vi "Generate Calibration Resists.vi"(1 "T Resolution":dbl=0.001 format="%.4f", 2 "End T":dbl=310.0 format="%.2f", 3 "Start T":dbl=1.0 format="%.2f", 4 "# of Points":i32=97) -> (0 "?":dbl[](array[numeric]) format="%.4f")   [LabVIEW 2020]
panel:
  # "Temperatures"
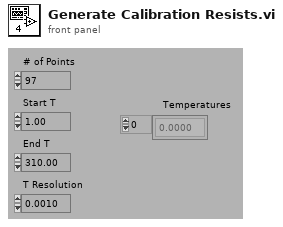
[diagram p1: front panel]
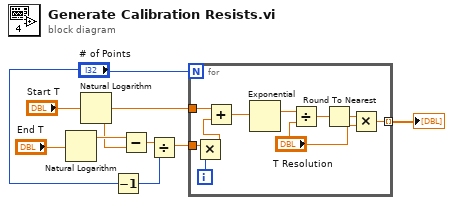
[diagram p0: block diagram]
diagram:
  n1 = Natural Logarithm(1:"End T") -> (0:w2:dbl)
  n2 = Natural Logarithm(1:"Start T") -> (0:w1:dbl)
  n3 = Decrement(x="# of Points") -> (x-1=w6:i32)
  n4 = Subtract(x=w2, y=w1) -> (x-y=w7:dbl)
  n5 = Divide(x=w7, y=w6) -> (x/y=w4:dbl)
  n6 = for {
    N: "# of Points" -> [_]
    tunnel: w1 -> [w19]
    tunnel: w4 -> [w17]
    tunnel: [w10] -> w3 mode=indexing
    i -> [w18]
    n7 = Multiply(x=w17, y=w18) -> (x*y=w16:dbl)
    n8 = Add(x=w19, y=w16) -> (x+y=w15:dbl)
    n9 = Exponential(1:w15) -> (0:w13:dbl)
    n10 = Divide(x=w13, y="T Resolution") -> (x/y=w12:dbl)
    n11 = Round To Nearest(number=w12) -> (nearest integer value=w11:dbl)
    n12 = Multiply(x=w11, y="T Resolution") -> (x*y=w10:dbl)
  }
  "?" <- w3
